vi "Create Frequency Steps Array.vi"(9 "Fine region centers":dbl[](array[numeric]), 10 "Leading steps to wait":i32=5, 11 "Spectrum Recorder Configuration":T1={"Start frequency"=500000.0, "End frequency"=2000000.0, "Coarse step"=100.0, "Step duration"=0.004, "Red Pitaya address"="192.168.1.100", "Open plot \non start"=FALSE, "Regions width"=2000.0, "Fine step"=1.0, "Pause between scans"=0.0, "Clear rgs on start"=FALSE, "Output amplitude"=1.0} {"Output amplitude" min=0.0 max=1.0 step=0.1 format="%#_6pV"; "Pause between scans" format="%#_6ps"; "Fine step" min=0.001 format="%#_6pHz"; "Regions width" format="%#_6pHz"; "Step duration" format="%#_6ps"; "Coarse step" format="%#_6pHz"; "End frequency" format="%#_6pHz"; "Start frequency" format="%#_6pHz"}) -> (3 "Steps":dbl[](array[numeric]) format="%#_8p")   [LabVIEW 2016]
uses:
  NHMFL_Core/Libraries/Red Pitaya/RP Core/Red Pitaya Transceiver Driver/Spectrum Configuration.ctl
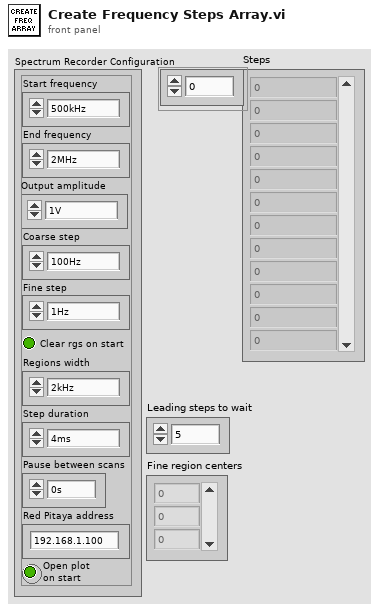
[diagram p1: front panel]
types:
  T1 = typedef "Spectrum Configuration.ctl" = cluster{"Start frequency":dbl, "End frequency":dbl, "Coarse step":dbl, "Step duration":dbl, "Red Pitaya address":string, "Open plot \non start":bool, "Regions width":dbl, "Fine step":dbl, "Pause between scans":dbl, "Clear rgs on start":bool, "Output amplitude":dbl}
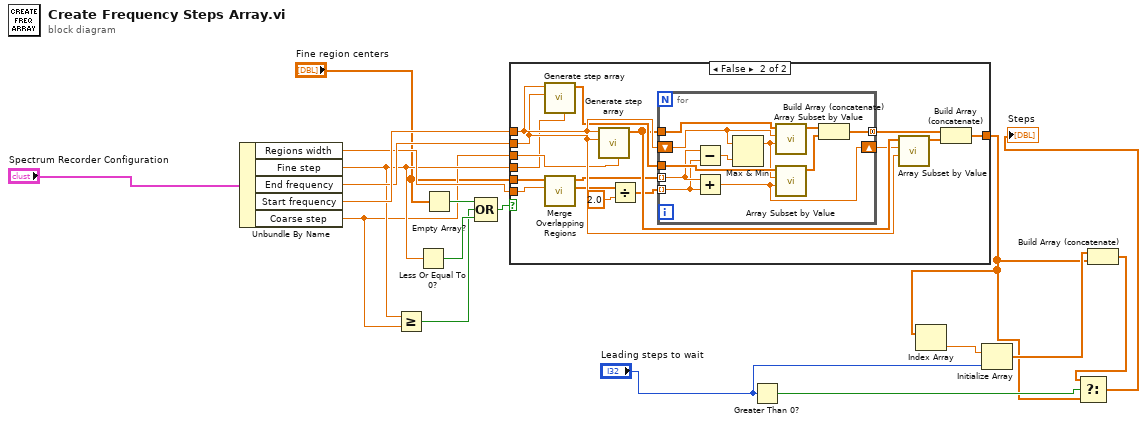
[diagram p0: block diagram]
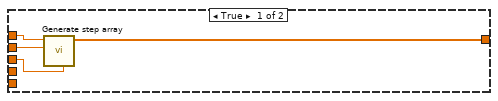
[diagram p2: hidden frame]
diagram:
  n1 = Unbundle By Name("Spectrum Recorder Configuration") -> ("Regions width"=w13:dbl, "Fine step"=w11:dbl, "End frequency"=w17:dbl, "Start frequency"=w18:dbl, "Coarse step"=w10:dbl)
  n2 = Greater Or Equal?(x=w11, y=w10) -> (x >= y?=w9:bool)
  n3 = Less Or Equal To 0?(x=w11) -> (x <= 0?=w12:bool)
  n4 = Empty Array?(array="Fine region centers") -> (empty?=w15:bool)
  n5 = Compound Arithmetic op=OR(w15, w9, w12) -> (w14:bool)
  n6 = case shown="False" w14 {
    tunnel: [w19 w31] -> w3
    tunnel: w17 -> [w21 w34]
    tunnel: w18 -> [w22 w38]
    tunnel: w10 -> [w20 w24]
    tunnel: w11 -> [_ w23]
    tunnel: "Fine region centers" -> [_ w27]
    tunnel: w13 -> [_ w30]
    frame True {
      n7 = call "Generate step array.vi"("Step"=w20, "End"=w21, "Start"=w22) -> ("Steps"=w19:dbl[])  [unwired: 8 in]
    }
    frame False {
      n8 = call "Generate step array.vi"("Step"=w23, "End"=w34, "Start"=w38) -> ("Steps"=w37:dbl[])  [unwired: 8 in]
      n9 = call "Merge Overlapping Regions.vi"("Regions width"=w30, "Region centers"=w27) -> ("Region widths out"=w28:dbl[], "Region centers out"=w26:dbl[])  [unwired: 8 in]
      n10 = call "Generate step array.vi"("Step"=w24, "End"=w34, "Start"=w38) -> ("Steps"=w36:dbl[])  [unwired: 8 in]
      n11 = Divide(x=w28, y=2.0) -> (x/y=w25:dbl[])
      n12 = for {
        tunnel: w26 -> [w47] mode=indexing
        tunnel: w36 -> [w49]
        tunnel: w25 -> [w46] mode=indexing
        shift-right: [w42] -> w35
        shift-left: w38 -> [w41]
        tunnel: w37 -> [w48]
        tunnel: [w43] -> w33 mode=concatenating
        n13 = Subtract(x=w47, y=w46) -> (x-y=w40:dbl)
        n14 = Add(x=w47, y=w46) -> (x+y=w42:dbl)
        n15 = Max & Min(x=w41, y=w40) -> (max(x,y)=w39:dbl)  [unwired: 1 out]
        n16 = call "Array Subset by Value.vi"("End"=w39, "Start"=w41, "Data"=w49) -> ("Data subset"=w45:dbl[])  [unwired: 8 in]
        n17 = call "Array Subset by Value.vi"("End"=w42, "Start"=w39, "Data"=w48) -> ("Data subset"=w44:dbl[])  [unwired: 8 in]
        n18 = Build Array (concatenate)(w45, w44) -> (w43:dbl[])
      }
      n19 = call "Array Subset by Value.vi"("End"=w34, "Start"=w35, "Data"=w36) -> ("Data subset"=w32:dbl[])  [unwired: 8 in]
      n20 = Build Array (concatenate)(w33, w32) -> (w31:dbl[])
    }
  }
  n21 = Greater Than 0?(x="Leading steps to wait") -> (x > 0?=w6:bool)
  n22 = Index Array(array=w3) -> (element=w8:dbl)  [unwired: 1 in]
  n23 = Initialize Array(w8, "Leading steps to wait") -> (w5:dbl[])
  n24 = Build Array (concatenate)(w5, w3) -> (w4:dbl[])
  n25 = Select(t=w4, s=w6, f=w3) -> (s? t:f=→"Steps":dbl[])
